vi "FGV_HovaCAL_Interface_MFC_Gase.vi"(6 "Aktion":T1, 8 "Fehler (Eingang, kein Fehler)":errorcluster, 10 "mfc Gasnamen in":string[](array[string]), 11 "mfc Gaslisten in":string[][](array[string])) -> (0 "Fehler (Ausgang)":errorcluster, 2 "mfc Gasnamen out":string[](array[string]), 3 "mfc Gaslisten out":string[][](array[string]))   [LabVIEW 2020, in "Linearisierung v2.lvlib" / "Gasteiler.lvlib" / "HovaCAL_Interface.lvlib" / "Kommunikation.lvlib"]
uses:
  Kommunikation.lvlib
  Aktion_FGV_HovaCAL_Interface_Gasliste.ctl
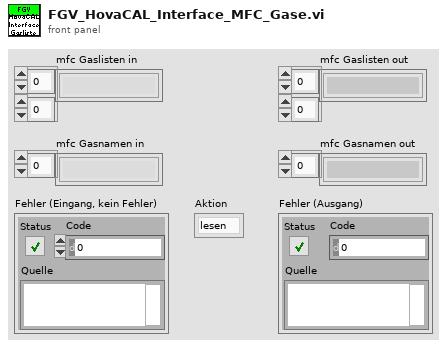
[diagram p1: front panel]
types:
  T1 = typedef "Linearisierung v2.lvlib/Gasteiler.lvlib/HovaCAL_Interface.lvlib/Kommunikation.lvlib/Aktion_FGV_HovaCAL_Interface_Gasliste.ctl" = enum16{"lesen", "setzen", "erstellen"}
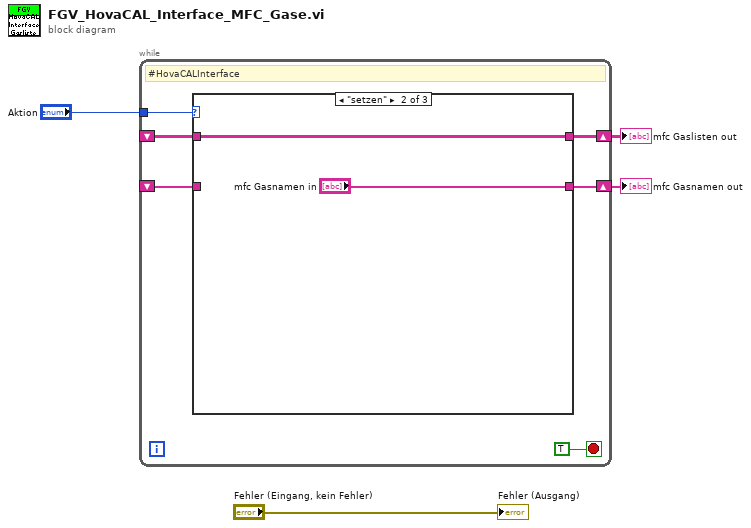
[diagram p0: block diagram]
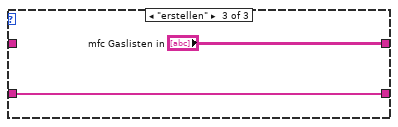
[diagram p3: hidden frame]
diagram:
  n1 = while {
    tunnel: "Aktion" -> [w9]
    shift-right: [w8] -> w3
    shift-left: _ -> [w7]
    shift-right: [w6] -> w2
    shift-left: _ -> [w5]
    stop <- TRUE stop-if-true
    # "#HovaCALInterface"
    n2 = case shown="\"setzen\"" w9 {
      tunnel: [w12 w14 "mfc Gaslisten in"] -> w8
      tunnel: w7 -> [w12 w14 _]
      tunnel: [w11 "mfc Gasnamen in" w15] -> w6
      tunnel: w5 -> [w11 _ w15]
      frame "lesen", Default {
      }
      frame "setzen" {
      }
      frame "erstellen" {
      }
    }
  }
  "mfc Gaslisten out" <- w3
  "mfc Gasnamen out" <- w2
  "Fehler (Ausgang)" <- "Fehler (Eingang, kein Fehler)"
